vi "GetRightClickMenu.vi"(0 "reference in":refnum<class "DqmhModuleDiagramGraph.lvclass">, 5 "error in (no error)":errorcluster) -> (14 "reference out":refnum<class "DqmhModuleDiagramGraph.lvclass">, 15 "Array":string[](array[string]), 16 "Found":bool, 19 "error out":errorcluster)   [LabVIEW 2014, in "DqmhModuleDiagramGraph.lvclass"]
doc: "GetRightClickMenu"
uses:
  <resource>/Framework/Providers/Open_GDS/UML/DqmhModuleDiagramGraph_class/DqmhModuleDiagramGraph.lvclass
  <resource>/Framework/Providers/Open_GDS/UML/DQMHModuleNode_class/DQMHModuleNode.lvclass
  <resource>/Framework/Providers/Open_GDS/UML/AbstractNode_class/AbstractNode.lvclass
  <resource>/Framework/Providers/Open_GDS/UML/Graph_class/Graph.lvclass
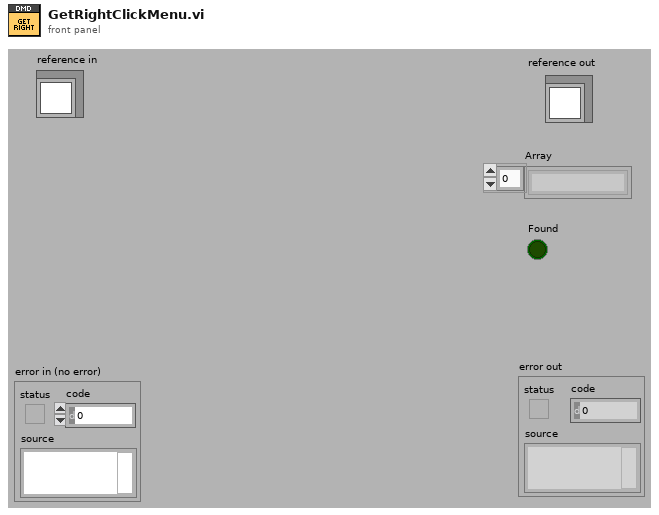
[diagram p1: front panel]
types:
  T1 = typedef "Graph.lvclass/ObjectAttributes.ctl" = cluster{"nodes":refnum<class "AbstractNode.lvclass">[], "edges":refnum<class "AbstractEdge.lvclass">[], "nodesToBeRemoved":refnum<class "AbstractNode.lvclass">[], "edgesToBeRemoved":refnum<class "AbstractEdge.lvclass">[], "needsLayout":bool, "LayoutNodes":refnum<class "AbstractNode.lvclass">[]}
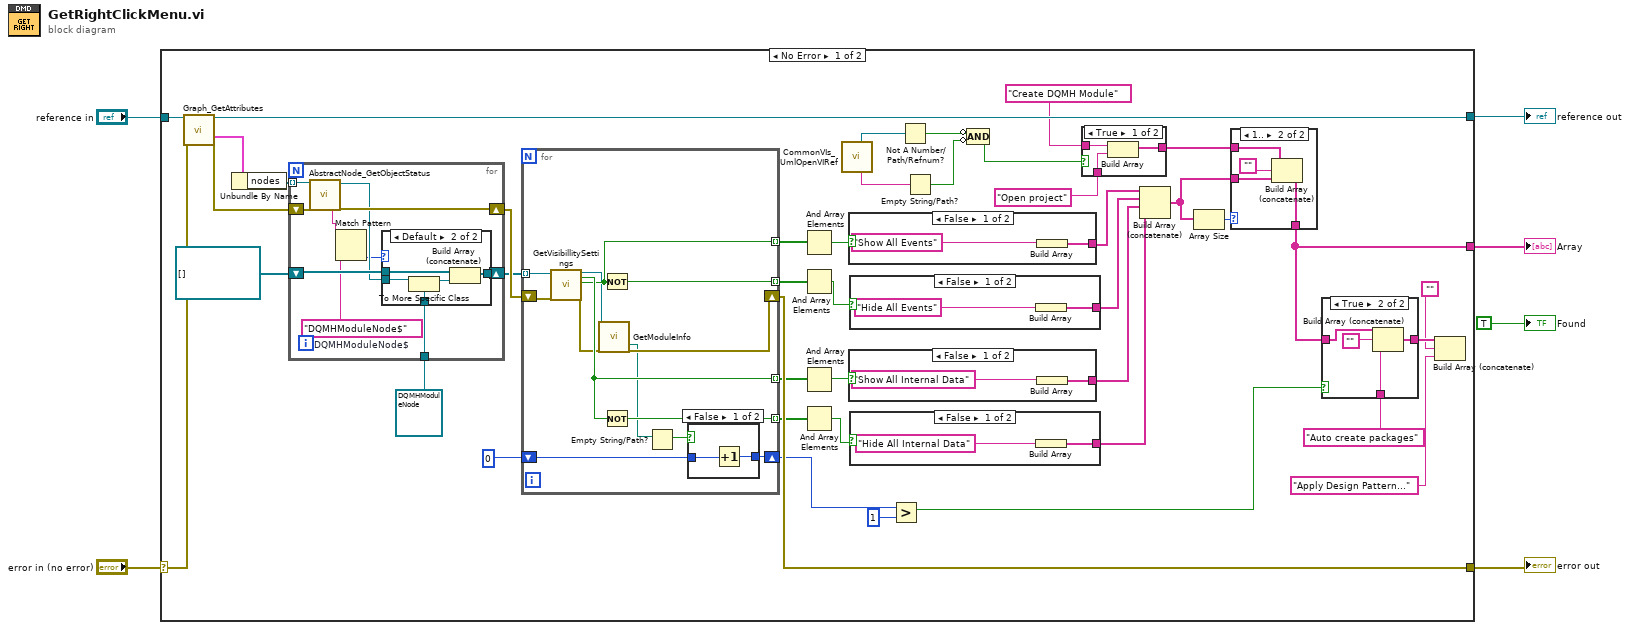
[diagram p0: block diagram]
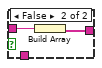
[diagram p3: hidden frame]
diagram:
  n1 = case shown="No Error" "error in (no error)" {
    selector: "error in (no error)" -> [w48 w104]
    tunnel: "reference in" -> [w47 w105]
    tunnel: [w42 w104] -> w4
    tunnel: [w46 w105] -> w3
    tunnel: [w8 _] -> w2
    frame No Error {
      n2 = call <resource>:"Graph_GetAttributes.vi"("reference in"=w47, "error in (no error)"=w48) -> ("reference out"=w46:refnum<class "DqmhModuleDiagramGraph.lvclass">, "Data"=w9:T1, "error out"=w43:errorcluster)  [unwired: 14 in, 1 out]
      n3 = Unbundle By Name(w9) -> ("nodes"=w19:refnum<class "AbstractNode.lvclass">[])
      n4 = for {
        shift-right: [w95] -> w44
        shift-left: w43 -> [w97]
        tunnel: w19 -> [w96] mode=indexing
        shift-right: [w92] -> w17
        shift-left: refnum<class "DQMHModuleNode.lvclass">[] [] -> [w94]
        tunnel: refnum<class "DQMHModuleNode.lvclass"> refnum ("DQMHModuleNode") -> [w89]
        w91 = "DQMHModuleNode$"  # DQMHModuleNode$
        n5 = call <resource>:"AbstractNode_GetObjectStatus.vi"("reference in"=w96, "error in (no error)"=w97) -> ("Class name"=w88:string, "reference out"=w93:refnum<class "AbstractNode.lvclass">, "error out"=w95:errorcluster)  [unwired: 15 out]
        n6 = Match Pattern(string=w88, regular expression=w91) -> (offset past match=w90:i32)  [unwired: 4 out]
        n7 = case shown="Default" w90 {
          tunnel: w94 -> [w98 w103]
          tunnel: w93 -> [_ w101]
          tunnel: [w98 w102] -> w92
          tunnel: w89 -> [_ w99]
          frame -1 {
          }
          frame Default {
            n8 = To More Specific Class(target class=w99, reference=w101) -> (specific class reference=w100:refnum<class "DQMHModuleNode.lvclass">)  [unwired: 1 in, 1 out]
            n9 = Build Array (concatenate)(w103, w100) -> (w102:refnum<class "DQMHModuleNode.lvclass">[])
          }
        }
      }
      n10 = for {
        tunnel: w17 -> [w84] mode=indexing
        shift-right: [w77] -> w42
        shift-left: w44 -> [w83]
        tunnel: [w80] -> w38 mode=indexing
        tunnel: [w79] -> w39 mode=indexing
        tunnel: [w81] -> w33 mode=indexing
        tunnel: [w82] -> w32 mode=indexing
        shift-right: [w72] -> w15
        shift-left: 0 ("y") -> [w73]
        n11 = call <resource>:"GetVisibillitySettings.vi"("reference in"=w84, "error in (no error)"=w83) -> ("reference out"=w75:refnum<class "DQMHModuleNode.lvclass">, "showAttribute"=w82:bool, "showMethods"=w79:bool, "error out"=w78:errorcluster)  [unwired: 14 in]
        n12 = call-dynamic "GetModuleInfo.vi"("reference in"=w75, "error in (no error)"=w78) -> ("ModulePath"=w76:path, "error out"=w77:errorcluster)  [unwired: 6 in, 10 out]
        n13 = Not(x=w79) -> (.not. x?=w80:bool)
        n14 = Not(x=w82) -> (.not. x?=w81:bool)
        n15 = Empty String/Path?(string/path=w76) -> (empty?=w74:bool)
        n16 = case shown="False" w74 {
          tunnel: w73 -> [w86 w87]
          tunnel: [w85 w87] -> w72
          frame False {
            n17 = Increment(x=w86) -> (x+1=w85:i32)
          }
          frame True {
          }
        }
      }
      n18 = And Array Elements(Boolean array=w39) -> (logical AND=w37:bool)
      n19 = And Array Elements(Boolean array=w38) -> (logical AND=w36:bool)
      n20 = And Array Elements(Boolean array=w32) -> (logical AND=w31:bool)
      n21 = And Array Elements(Boolean array=w33) -> (logical AND=w30:bool)
      n22 = call <resource>:"CommonVIs_UmlOpenVIRef.vi"() -> ("ProjectNameOut"=w24:string, "AppRefOut"=w25:refnum<vi>)  [unwired: 4 in, 6 out]
      n23 = case shown="False" w37 {
        tunnel: [w71 _] -> w41
        frame False {
          n24 = Build Array("Show All Events") -> (w71:string[])
        }
        frame True {
        }
      }
      n25 = case shown="False" w31 {
        tunnel: [w62 _] -> w29
        frame False {
          n26 = Build Array("Show All Internal Data") -> (w62:string[])
        }
        frame True {
        }
      }
      n27 = case shown="False" w36 {
        tunnel: [w69 _] -> w40
        frame False {
          n28 = Build Array("Hide All Events") -> (w69:string[])
        }
        frame True {
        }
      }
      n29 = case shown="False" w30 {
        tunnel: [w60 _] -> w28
        frame False {
          n30 = Build Array("Hide All Internal Data") -> (w60:string[])
        }
        frame True {
        }
      }
      n31 = Greater?(x=w15, y=1) -> (0:w14:bool)
      n32 = Not A Number/Path/Refnum?(number/path/refnum=w25) -> (NaN/Path/Refnum?=w23:bool)
      n33 = Empty String/Path?(string/path=w24) -> (empty?=w22:bool)
      n34 = Compound Arithmetic op=AND(invert w23, invert w22) -> (w21:bool)
      n35 = case shown="True" w21 {
        tunnel: "Create DQMH Module" -> [w56 w58]
        tunnel: [w55 w57] -> w26
        tunnel: "Open project" ("element") -> [w54 _]
        frame True {
          n36 = Build Array(w56, w54) -> (w55:string[])
        }
        frame False {
          n37 = Build Array(w58) -> (w57:string[])
        }
      }
      n38 = Build Array (concatenate)(w41, w40, w29, w28) -> (w35:string[])
      n39 = Array Size(array=w35) -> (size(s)=w34:i32)
      n40 = case shown="1.." w34 {
        tunnel: [w63 w67] -> w8
        tunnel: w26 -> [w63 w66]
        tunnel: w35 -> [_ w65]
        frame Default {
        }
        frame 1.. {
          n41 = Build Array (concatenate)(w66, "", w65) -> (w67:string[])
        }
      }
      n42 = case shown="True" w14 {
        tunnel: w8 -> [w49 w51]
        tunnel: [w49 w52] -> w12
        tunnel: "Auto create packages" -> [_ w50]
        frame False {
        }
        frame True {
          n43 = Build Array (concatenate)(w51, "", w50) -> (w52:string[])
        }
      }
      n44 = Build Array (concatenate)(w12, "", "Apply Design Pattern..." ("element")) -> ()  [unwired: 1 out]
    }
    frame Error {
    }
  }
  "reference out" <- w3
  "error out" <- w4
  "Array" <- w2
  "Found" <- TRUE ("Found")
